vi "Setup.vi"(6 "Config in":T1, 7 "DisplayFilter":u8(ring)=7 items=["K_CHAN_R", "K_CHAN_W", "K_CHAN_RW", "K_CHAN_VOLT", "K_CHAN_FAULT", "K_ALL", "K_CUSTOM", "K_CHAN_R_VIS", "K_CHAN_W_VIS", "K_CHAN_RW_VIS", "K_CHAN_VOLT_VIS", "K_CHAN_FAULT_VIS"], 8 "error in (no error)":errorcluster, 9 "Caption":string, 10 "nodePath":string, 11 "NIVS.System Definition Root":refnum<k24>) -> (0 "error out":errorcluster, 1 "Caption out":string, 2 "Cancel?":bool, 3 "Selected Item":T2, 4 "List out":T1)   [LabVIEW 2015, in "Workspace.Obejct.Radio.lvlib"]
uses:
  Workspace.Obejct.Radio.lvlib
  NationalInstruments.VeriStand.SystemStorageUI
  NationalInstruments.VeriStand.SystemStorage
  <vilib>/NI Veristand/UI Controls/Single Node Browser/Node Ref.ctl
  Types/Config.ctl
  Types/Setup.StateVariables.ctl
  <vilib>/NI Veristand/UI Controls/Single Node Browser/Net Event Data.ctl
  <vilib>/NI Veristand/UI Controls/Single Node Browser/Net Event.ctl
  <vilib>/Utility/miscctls.llb/LVRowAndColumnTypeDef.ctl
  NationalInstruments.VeriStand
  <vilib>/NI Veristand/UI Controls/Single Node Browser/NI_VS UI Single Node Browser.lvlib
panel:
  in  "AutoUpdate":bool
  in  "Cancel":bool
  in  "OK":bool
  in  "Value":i64
  in  "Name":string
  in  "Text Value Pairing":i32(listbox)
  in  "Single Node Browser":refnum<k24>(container)
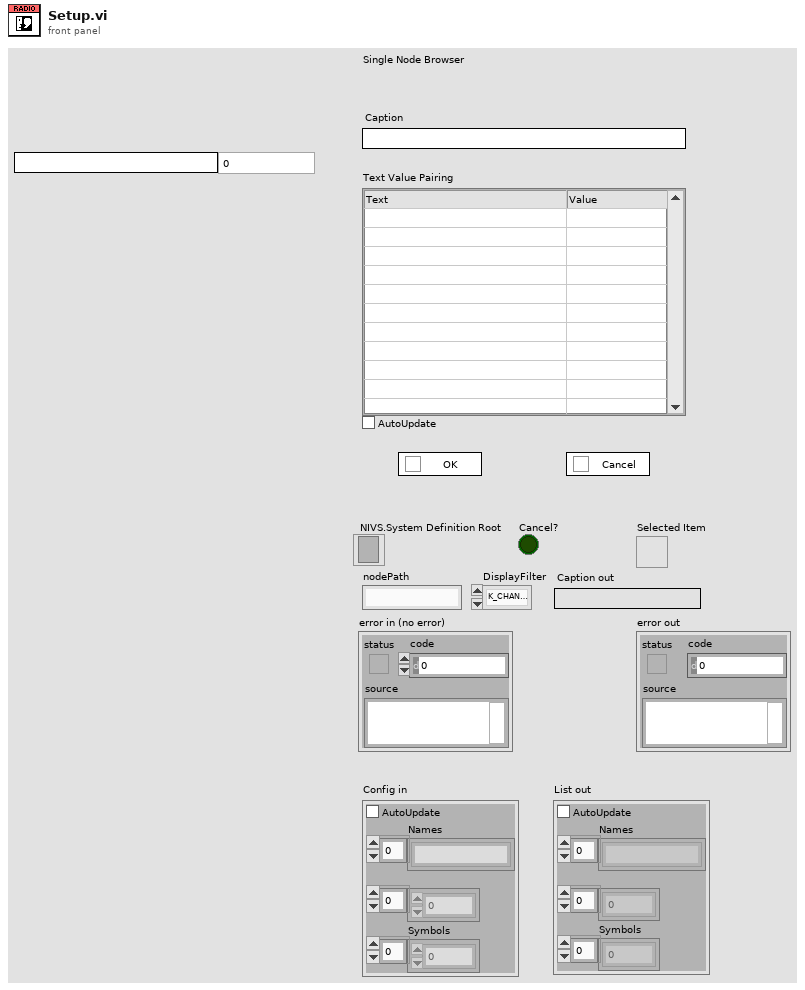
[diagram p1: front panel]
types:
  T1 = typedef "Workspace.Obejct.Radio.lvlib/Config.ctl" = cluster{"AutoUpdate":bool, "Names":string[], "Values":dbl[], "Symbols":i32[]}
  T2 = typedef "NI_VS UI Single Node Browser.lvlib/Node Ref.ctl" = refnum<k24>
  T3 = typedef "Workspace.Obejct.Radio.lvlib/Setup.StateVariables.ctl" = cluster{"UI.TextValuePairing":refnum<vi>, "UI.AutoUpdate":refnum<vi>, "UI.Name":refnum<vi>, "UI.Value":refnum<vi>, "UI.Caption":refnum<vi>, "UI.Events":refnum<event-registration>, "Config":T1, "NIVS.SystemDefinitionRoot":refnum<k24>, "NIVS.SingleNodeBrowser":refnum<k24>, "NIVS.NodePath":string, "NIVS.DisplayFilter":u8, "NIVS.Node":refnum<k24>, "Cache.Row":i32, "Cache.CellPosition":T4}
  T4 = typedef "LVRowAndColumnTypeDef.ctl" = cluster{"Row":i32, "Column":i32}
  T5 = enum8{"Enabled", "Disabled", "Disabled and Grayed Out"}
  T6 = typedef "LVPoint32TypeDef.ctl" = cluster{"Horizontal":i32, "Vertical":i32}
  T7 = typedef "LVPositionTypeDef.ctl" = cluster{"Left":i32, "Top":i32}
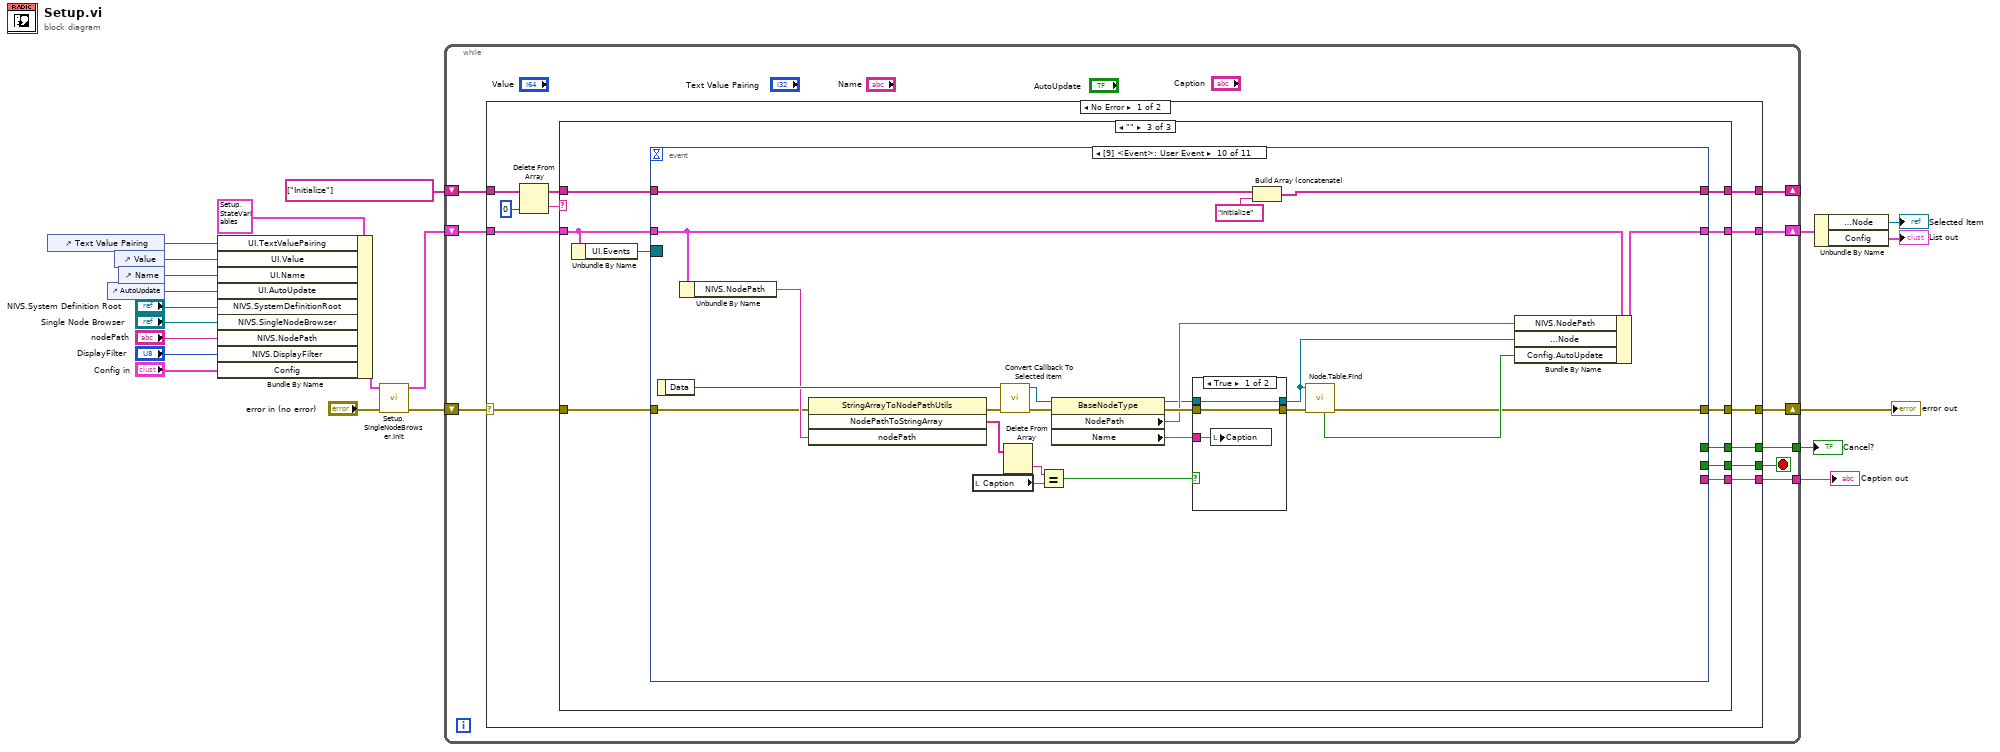
[diagram p0: block diagram]
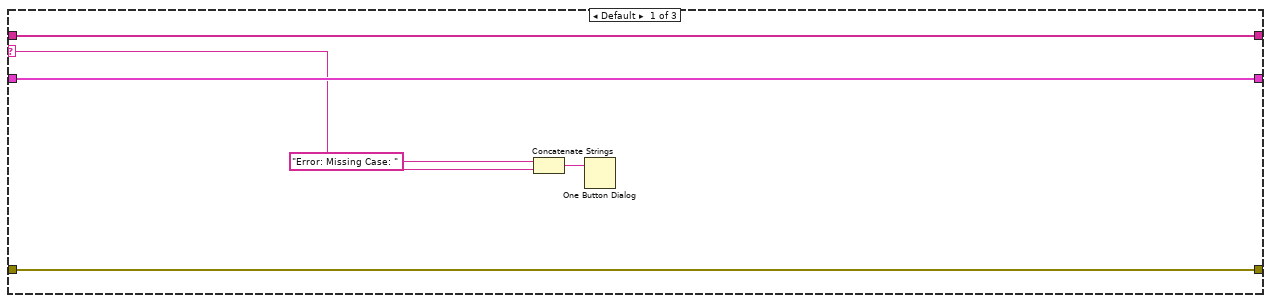
[diagram p2: hidden frame]
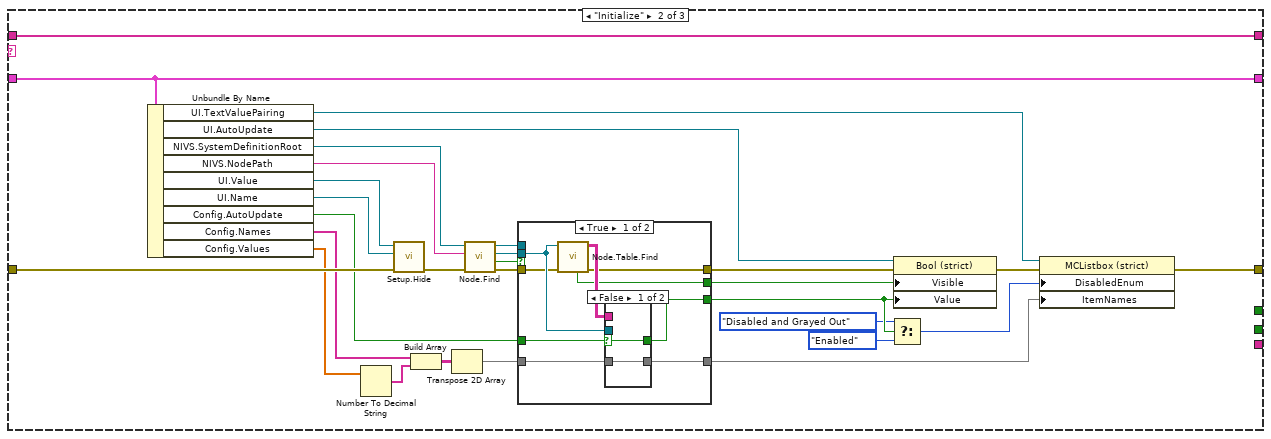
[diagram p3: hidden frame]
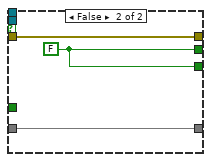
[diagram p5: hidden frame]
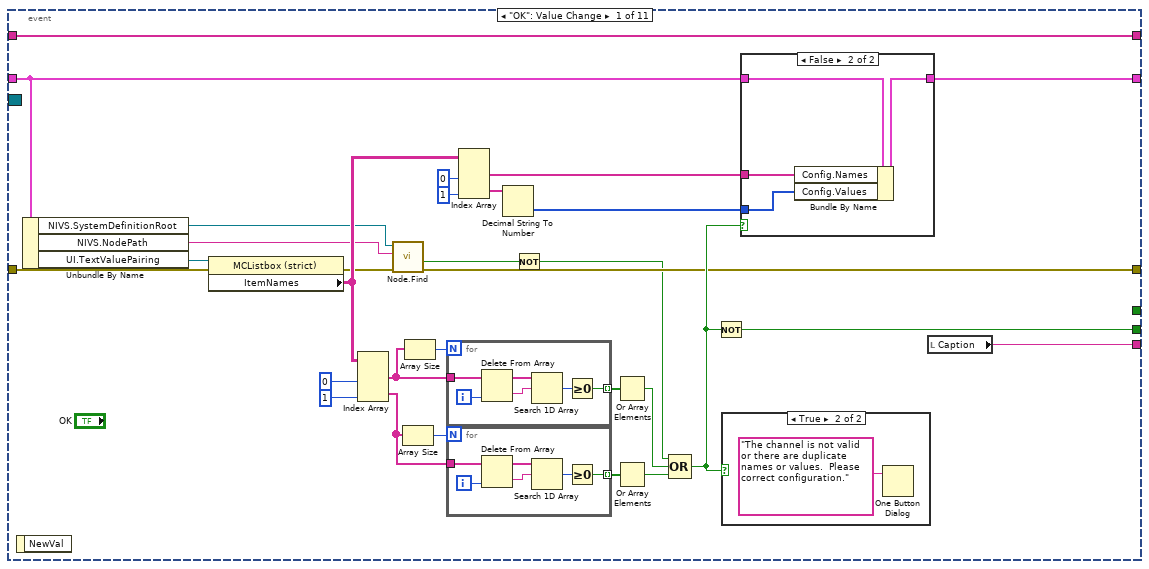
[diagram p6: hidden frame]
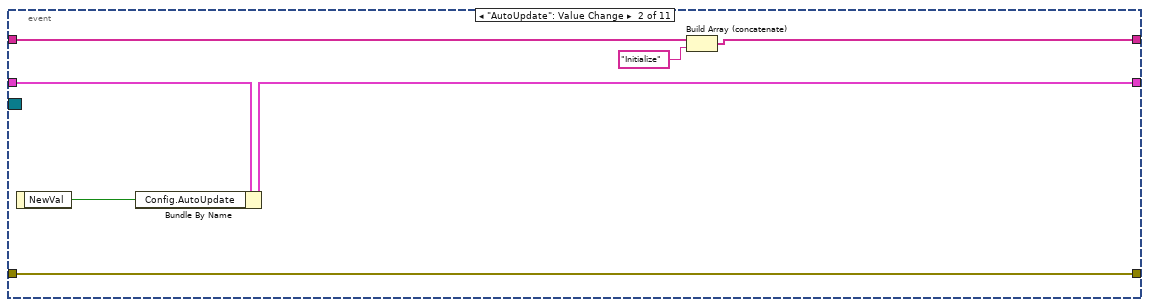
[diagram p9: hidden frame]
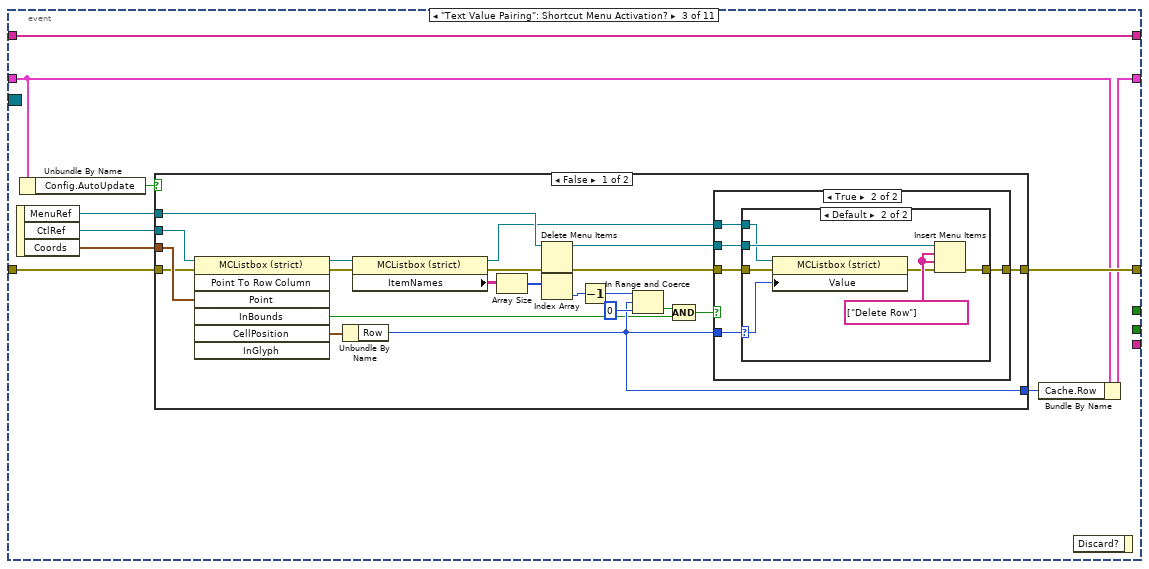
[diagram p10: hidden frame]
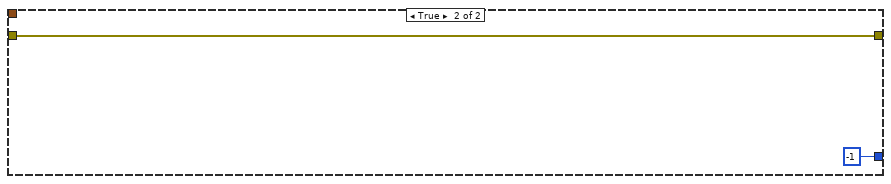
[diagram p13: hidden frame]
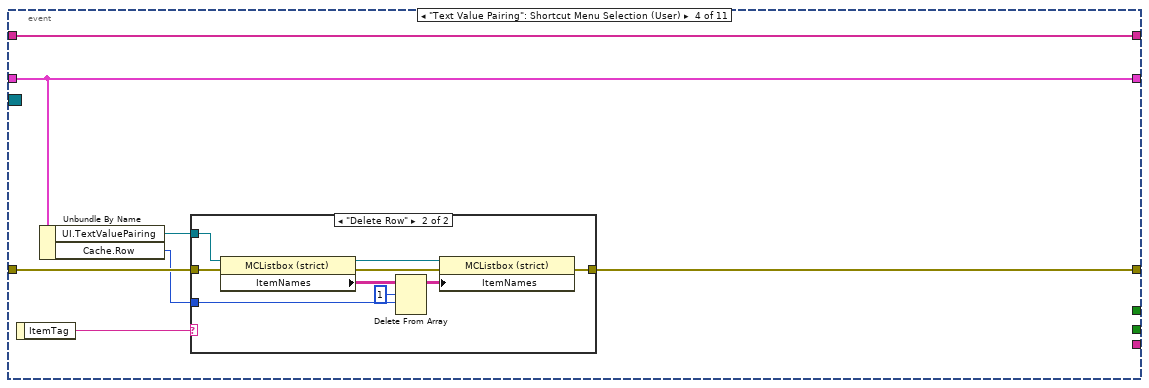
[diagram p14: hidden frame]
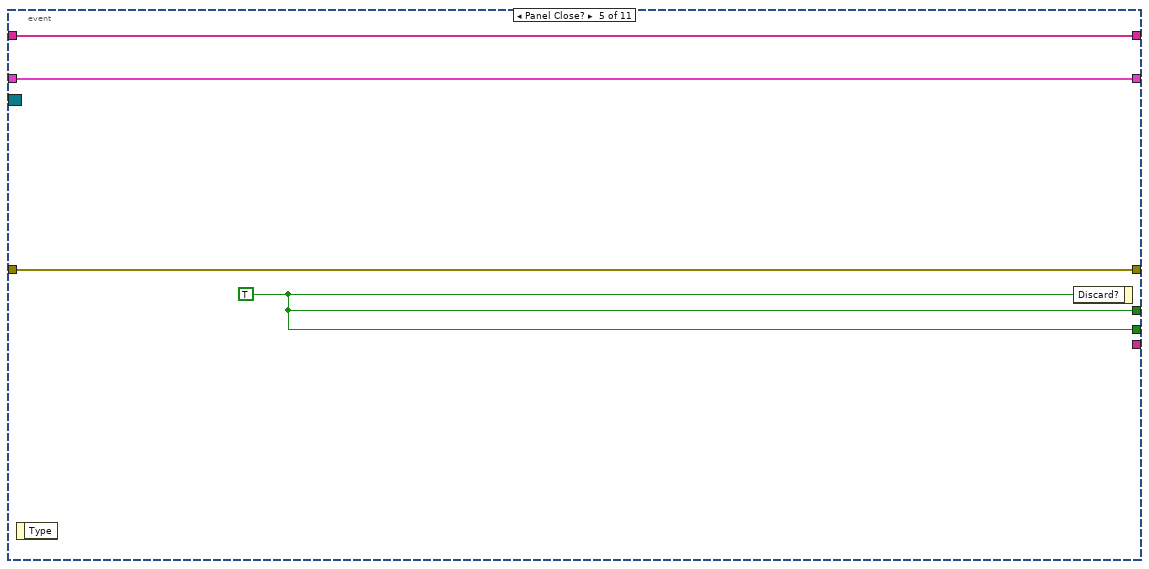
[diagram p16: hidden frame]
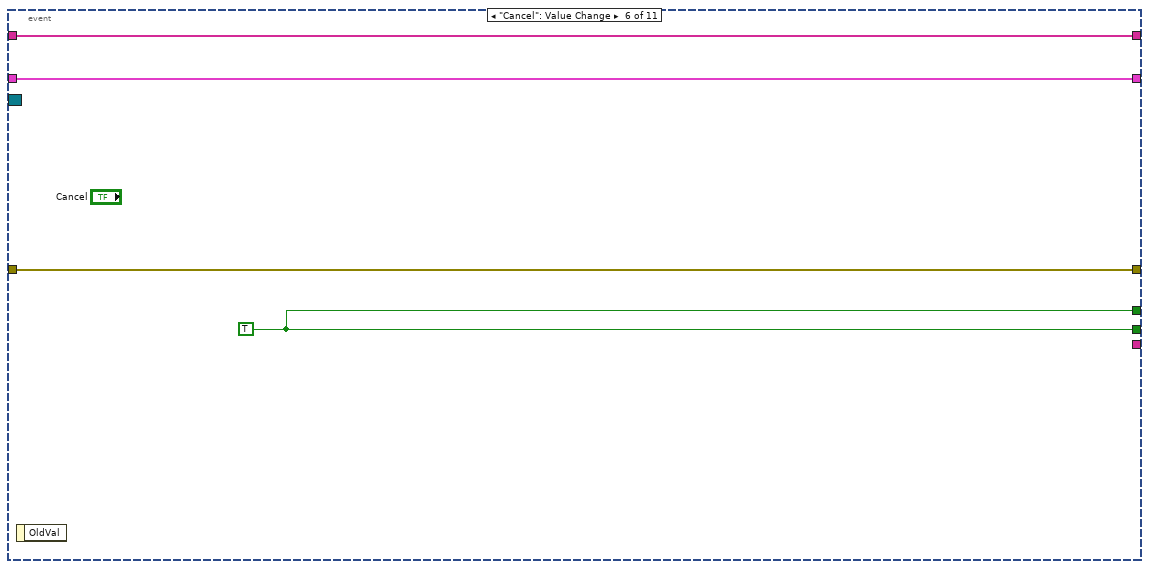
[diagram p17: hidden frame]
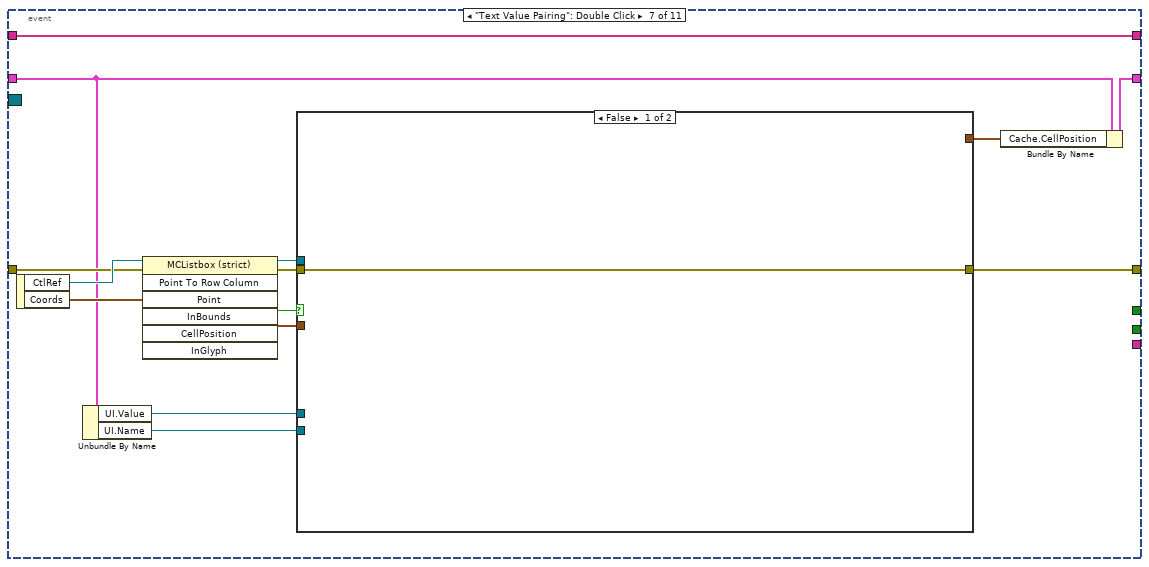
[diagram p18: hidden frame]
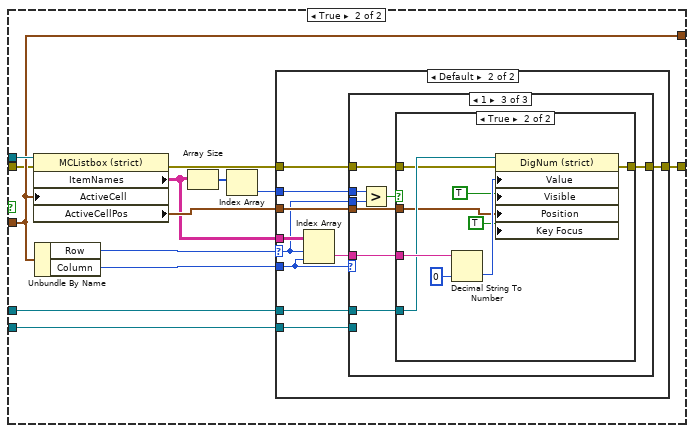
[diagram p19: hidden frame]
diagram:
  n1 = control-ref of="Text Value Pairing"() -> (w20:refnum<vi>)
  n2 = control-ref of="AutoUpdate"() -> (w17:refnum<vi>)
  n3 = control-ref of="Value"() -> (w19:refnum<vi>)
  n4 = control-ref of="Name"() -> (w18:refnum<vi>)
  n5 = Bundle By Name(cluster=T3 {"UI.TextValuePairing"=refnum, "UI.AutoUpdate"=refnum, "UI.Name"=refnum, "UI.Value"=refnum, "UI.Caption"=refnum, "UI.Events"=refnum, "Config"={"AutoUpdate"=FALSE, "Names"=[], "Values"=[], "Symbols"=[]}, "NIVS.SystemDefinitionRoot"=refnum, "NIVS.SingleNodeBrowser"=refnum, "NIVS.NodePath"="", "NIVS.DisplayFilter"=7, "NIVS.Node"=refnum, "Cache.Row"=0, "Cache.CellPosition"={"Row"=0, "Column"=0}} ("Cluster"), "UI.TextValuePairing"=w20, "UI.Value"=w19, "UI.Name"=w18, "UI.AutoUpdate"=w17, "NIVS.SystemDefinitionRoot"="NIVS.System Definition Root", "NIVS.SingleNodeBrowser"="Single Node Browser", "NIVS.NodePath"="nodePath", "NIVS.DisplayFilter"="DisplayFilter", "Config"="Config in") -> (w11:T3)
  n6 = call "Setup.SingleNodeBrowser.Init.vi"("error in (no error)"="error in (no error)", "Variables"=w11) -> ("error out"=w10:errorcluster, "Cluster out"=w9:T3)  [unwired: 8 in]
  n7 = while {
    shift-right: [w29] -> w5
    shift-left: w10 -> [w26]
    shift-right: [w27] -> w4
    shift-left: w9 -> [w28]
    shift-right: [w24] -> _
    shift-left: string[] ["Initialize"] -> [w25]
    tunnel: [w23] -> w6
    tunnel: [w22] -> w1
    stop <- w30 stop-if-true
    n8 = case shown="No Error" w26 {
      selector: w26 -> [w38 w399]
      tunnel: [w42 _] -> w30
      tunnel: [w41 w398] -> w29
      tunnel: w28 -> [w40 w402]
      tunnel: [w39 w402] -> w27
      tunnel: w25 -> [w36 w401]
      tunnel: [w33 w401] -> w24
      tunnel: [w32 _] -> w23
      tunnel: [w31 _] -> w22
      frame No Error {
        n9 = Delete From Array(array=w36, index=0) -> (deleted portion=w35:string, array with subset deleted=w34:string[])  [unwired: 1 in]
        n10 = case shown="\"\"" w35 {
          selector: w35 -> [w45 _ _]
          tunnel: [_ _ w102] -> w42
          tunnel: [w47 w60 w100] -> w41
          tunnel: w40 -> [w48 w50 w95]
          tunnel: [w48 w50 w99] -> w39
          tunnel: w38 -> [w47 w77 w103]
          tunnel: w34 -> [w46 w49 w97]
          tunnel: [w46 w49 w98] -> w33
          tunnel: [_ _ w101] -> w32
          tunnel: [_ _ w96] -> w31
          frame Default {
            n11 = Concatenate Strings("Error: Missing Case: " ("string"), w45) -> (w44:string)
            n12 = One Button Dialog(message=w44) -> ()  [unwired: 1 in, 1 out]
          }
          frame "Initialize" {
            n13 = Unbundle By Name(w50) -> ("UI.TextValuePairing"=w61:refnum<vi>, "UI.AutoUpdate"=w62:refnum<vi>, "NIVS.SystemDefinitionRoot"=w63:refnum<k24>, "NIVS.NodePath"=w64:string, "UI.Value"=w75:refnum<vi>, "UI.Name"=w76:refnum<vi>, "Config.AutoUpdate"=w53:bool, "Config.Names"=w51:string[], "Config.Values"=w52:dbl[])
            n14 = Number To Decimal String(number=w52) -> (decimal integer string=w70:string[])  [unwired: 1 in]
            n15 = call "Setup.Hide.vi"("error in (no error)"=w77, "Name"=w76, "Value"=w75) -> ("error out"=w67:errorcluster)  [unwired: 8 in]
            n16 = Build Array(w51, w70) -> (w69:string[][])
            n17 = Transpose 2D Array(2D array=w69) -> (transposed array=w68:string[][])
            n18 = call "Node.Find.vi"("error in (no error)"=w67, "nodePath"=w64, "System Def Root"=w63) -> ("error out"=w74:errorcluster, "FindNode"=w73:bool, "Node"=w72:refnum<k24>, "System Def Root"=w71:refnum<k24>)  [unwired: 5 in]
            n19 = case shown="True" w73 {
              tunnel: [w79 w91] -> w66
              tunnel: w71 -> [_ _]
              tunnel: w74 -> [w78 w91]
              tunnel: w72 -> [w82 _]
              tunnel: w53 -> [w84 _]
              tunnel: [w83 w93] -> w57
              tunnel: [w80 w93] -> w58
              tunnel: [w86 w92] -> w59
              tunnel: w68 -> [w85 w92]
              frame True {
                n20 = call "Node.Table.Find.vi"("error in (no error)"=w78, "Node"=w82) -> ("error out"=w79:errorcluster, "Items"=w81:string[][], "Found?"=w80:bool)  [unwired: 5 in, 2 out]
                n21 = case shown="False" w84 {
                  selector: w84 -> [w87 w90]
                  tunnel: w82 -> [_ _]
                  tunnel: [w88 w89] -> w86
                  tunnel: w85 -> [w88 _]
                  tunnel: [w87 w90] -> w83
                  tunnel: w81 -> [_ w89]
                  frame False {
                  }
                  frame True {
                  }
                }
              }
              frame False {
                w93 = FALSE ("AliasView")
              }
            }
            n22 = Select(t=T5."Disabled and Grayed Out" ("Disabled"), s=w57, f=T5."Enabled" ("Disabled")) -> (s? t:f=w54:T5)
            n23 = property class="Bool (strict)"(reference=w62, error in=w66, "Visible"=w58, "Value"=w57) -> (error out=w65:errorcluster)  [unwired: 1 out]
            n24 = property class="MCListbox (strict)"(reference=w61, error in=w65, "DisabledEnum"=w54, "ItemNames"=w59) -> (error out=w60:errorcluster)  [unwired: 1 out]
          }
          frame "" {
            n25 = Unbundle By Name(w95) -> ("UI.Events"=w94:refnum<event-registration>)
            n26 = event shown="[9] <Event>: User Event" {
              selector: w94 -> [_ _ _ _ _ _ _ _ _ _ _]
              dyn-events: _ -> [_ _ _ _ _ _ _ _ _ _ _]
              timeout: _ -> [_ _ _ _ _ _ _ _ _ _ _]
              tunnel: [w121 _ _ _ w226 w230 _ _ _ _ _] -> w102
              tunnel: w103 -> [w133 w155 w165 w211 w225 w229 w237 w324 w363 w375 w396]
              tunnel: [w108 w155 w168 w210 w225 w229 w238 w318 w353 w367 w397] -> w100
              tunnel: [_ _ _ _ w226 w230 _ _ _ _ _] -> w101
              tunnel: [w132 _ _ _ _ _ _ _ _ _ _] -> w96
              tunnel: [w112 w152 w159 w208 w224 w228 w234 w309 w351 w380 w394] -> w99
              tunnel: w95 -> [w113 w153 w161 w208 w224 w228 w233 w309 w351 w378 w394]
              tunnel: [w120 w157 w163 w209 w223 w227 w236 w310 w352 w366 w395] -> w98
              tunnel: w97 -> [w120 w158 w163 w209 w223 w227 w236 w310 w352 w381 w395]
              event "OK": Value Change {
                n27 = event-data() -> ()  [unwired: 1 in, 1 out]
                n28 = Unbundle By Name(w113) -> ("NIVS.SystemDefinitionRoot"=w106:refnum<k24>, "NIVS.NodePath"=w107:string, "UI.TextValuePairing"=w119:refnum<vi>)
                n29 = property class="MCListbox (strict)"(reference=w119, error in=w133) -> (error out=w109:errorcluster, "ItemNames"=w115:string[][])  [unwired: 1 out]
                n30 = Index Array(array=w115, index (col) #1=0 ("disabled index (col)"), index (col) #2=1 ("index (col)")) -> (element #1=w128:string[], element #2=w124:string[])  [unwired: 2 in]
                n31 = call "Node.Find.vi"("error in (no error)"=w109, "nodePath"=w107, "System Def Root"=w106) -> ("error out"=w108:errorcluster, "FindNode"=w105:bool)  [unwired: 5 in, 2 out]
                n32 = Array Size(array=w124) -> (size(s)=w125:i32)
                n33 = Array Size(array=w128) -> (size(s)=w129:i32)
                n34 = for {
                  N: w129 -> [_]
                  tunnel: w128 -> [w151]
                  tunnel: [w146] -> w127 mode=indexing
                  i -> [w150]
                  n35 = Delete From Array(array=w151, index=w150) -> (deleted portion=w148:string, array with subset deleted=w149:string[])  [unwired: 1 in]
                  n36 = Search 1D Array(1D array=w149, element=w148) -> (index of element=w147:i32)  [unwired: 1 in]
                  n37 = Greater Or Equal To 0?(x=w147) -> (x >= 0?=w146:bool)
                }
                n38 = for {
                  N: w125 -> [_]
                  tunnel: w124 -> [w145]
                  tunnel: [w140] -> w123 mode=indexing
                  i -> [w144]
                  n39 = Delete From Array(array=w145, index=w144) -> (deleted portion=w142:string, array with subset deleted=w143:string[])  [unwired: 1 in]
                  n40 = Search 1D Array(1D array=w143, element=w142) -> (index of element=w141:i32)  [unwired: 1 in]
                  n41 = Greater Or Equal To 0?(x=w141) -> (x >= 0?=w140:bool)
                }
                n42 = Index Array(array=w115, index (col) #1=0 ("disabled index (col)"), index (col) #2=1 ("index (col)")) -> (element #1=w110:string[], element #2=w116:string[])  [unwired: 2 in]
                n43 = Decimal String To Number(string=w116) -> (number=w111:i32[])  [unwired: 2 in, 1 out]
                n44 = Not(x=w105) -> (.not. x?=w104:bool)
                n45 = Or Array Elements(Boolean array=w127) -> (logical OR=w126:bool)
                n46 = Or Array Elements(Boolean array=w123) -> (logical OR=w122:bool)
                n47 = Compound Arithmetic op=OR(w104, w126, w122) -> (w114:bool)
                n48 = Not(x=w114) -> (.not. x?=w121:bool)
                n49 = case shown="True" w114 {
                  frame False {
                  }
                  frame True {
                    n50 = One Button Dialog(message="The channel is not valid or there are duplicate names or values.  Please correct configuration.") -> ()  [unwired: 1 in, 1 out]
                  }
                }
                n51 = case shown="False" w114 {
                  tunnel: w113 -> [w134 w138]
                  tunnel: [w134 w137] -> w112
                  tunnel: w111 -> [_ w136]
                  tunnel: w110 -> [_ w135]
                  frame True {
                  }
                  frame False {
                    n52 = Bundle By Name(cluster=w138, "Config.Names"=w135, "Config.Values"=w136) -> (w137:T3)
                  }
                }
                n53 = local read "Caption"() -> (w132:string)
              }
              event "AutoUpdate": Value Change {
                n54 = event-data() -> ("NewVal"=w154:bool)  [unwired: 1 in]
                n55 = Bundle By Name(cluster=w153, "Config.AutoUpdate"=w154) -> (w152:T3)
                n56 = Build Array (concatenate)(w158, "Initialize") -> (w157:string[])
              }
              event "Text Value Pairing": Shortcut Menu Activation? {
                n57 = event-data() -> ("MenuRef"=w164:refnum<k9>, "CtlRef"=w167:refnum<vi>, "Coords"=w166:T6)  [unwired: 1 in]
                n58 = Unbundle By Name(w161) -> ("Config.AutoUpdate"=w162:bool)
                n59 = case shown="False" w162 {
                  tunnel: [w189 w205] -> w168
                  tunnel: w167 -> [w188 _]
                  tunnel: w166 -> [w187 _]
                  tunnel: w165 -> [w186 w205]
                  tunnel: [w177 -1 ("Row")] -> w160
                  tunnel: w164 -> [w171 _]
                  frame False {
                    n60 = invoke class="MCListbox (strict)" method="Point To Row Column"(reference=w188, error in=w186, "Point"=w187) -> (reference out=w184:refnum<vi>, error out=w183:errorcluster, "InBounds"=w175:bool, "CellPosition"=w185:T4)  [unwired: 4 in, 3 out]
                    n61 = Unbundle By Name(w185) -> ("Row"=w177:i32)
                    n62 = property class="MCListbox (strict)"(reference=w184, error in=w183) -> (reference out=w169:refnum<vi>, error out=w173:errorcluster, "ItemNames"=w182:string[][])
                    n63 = Array Size(array=w182) -> (size(s)=w181:i32[])
                    n64 = Delete Menu Items(6:w173, 9:w171) -> (0:w172:errorcluster, 3:w170:refnum<k9>)  [unwired: 2 in]
                    n65 = Index Array(array=w181) -> (element=w180:i32)  [unwired: 1 in]
                    n66 = Decrement(x=w180) -> (x-1=w179:i32)
                    n67 = In Range and Coerce(upper limit=w179, x=w177, lower limit=0) -> (In Range?=w176:bool)  [unwired: 1 out]
                    n68 = Compound Arithmetic op=AND(w176, w175) -> (w174:bool)
                    n69 = case shown="True" w174 {
                      tunnel: w170 -> [_ w195]
                      tunnel: [w190 w194] -> w189
                      tunnel: w172 -> [w190 w193]
                      tunnel: w177 -> [_ w192]
                      tunnel: w169 -> [_ w191]
                      frame False {
                      }
                      frame True {
                        n70 = case shown="Default" w192 {
                          selector: w192 -> [_ w197]
                          tunnel: w195 -> [_ w201]
                          tunnel: [w196 w203] -> w194
                          tunnel: w193 -> [w196 w200]
                          tunnel: w191 -> [_ w198]
                          frame -1 {
                          }
                          frame Default {
                            w202 = string[] ["Delete Row"] ("item names")
                            n71 = property class="MCListbox (strict)"(reference=w198, error in=w200, "Value"=w197) -> (error out=w199:errorcluster)  [unwired: 1 out]
                            n72 = Insert Menu Items(6:w199, 7:w202, 8:w202, 9:w201) -> (0:w203:errorcluster)  [unwired: 2 in, 2 out]
                          }
                        }
                      }
                    }
                  }
                  frame True {
                  }
                }
                n73 = Bundle By Name(cluster=w161, "Cache.Row"=w160) -> (w159:T3)
                n74 = event-data() -> ()  [unwired: 2 in, 1 out]
              }
              event "Text Value Pairing": Shortcut Menu Selection (User) {
                n75 = event-data() -> ("ItemTag"=w212:string)  [unwired: 1 in]
                n76 = Unbundle By Name(w208) -> ("UI.TextValuePairing"=w206:refnum<vi>, "Cache.Row"=w207:i32)
                n77 = case shown="\"Delete Row\"" w212 {
                  tunnel: w211 -> [w213 w222]
                  tunnel: w207 -> [_ w216]
                  tunnel: [w213 w215] -> w210
                  tunnel: w206 -> [_ w214]
                  frame "False", Default {
                  }
                  frame "Delete Row" {
                    n78 = property class="MCListbox (strict)"(reference=w214, error in=w222) -> (reference out=w220:refnum<vi>, error out=w221:errorcluster, "ItemNames"=w219:string[][])
                    n79 = Delete From Array(array=w219, length=1, index (row)=w216) -> (array with subset deleted=w218:string[][])  [unwired: 1 in, 1 out]
                    n80 = property class="MCListbox (strict)"(reference=w220, error in=w221, "ItemNames"=w218) -> (error out=w215:errorcluster)  [unwired: 1 out]
                  }
                }
              }
              event Panel Close? {
                w226 = TRUE ("Discard?")
                n81 = event-data() -> ()  [unwired: 1 in, 1 out]
                n82 = event-data("Discard?"=w226) -> ()  [unwired: 1 in, 1 out]
              }
              event "Cancel": Value Change {
                w230 = TRUE ("Discard?")
                n83 = event-data() -> ()  [unwired: 1 in, 1 out]
              }
              event "Text Value Pairing": Double Click {
                n84 = event-data() -> ("CtlRef"=w244:refnum<vi>, "Coords"=w243:T6)  [unwired: 1 in]
                n85 = Unbundle By Name(w233) -> ("UI.Value"=w231:refnum<vi>, "UI.Name"=w232:refnum<vi>)
                n86 = invoke class="MCListbox (strict)" method="Point To Row Column"(reference=w244, error in=w237, "Point"=w243) -> (reference out=w242:refnum<vi>, error out=w239:errorcluster, "InBounds"=w240:bool, "CellPosition"=w241:T4)  [unwired: 4 in, 3 out]
                n87 = case shown="False" w240 {
                  tunnel: w241 -> [_ w254]
                  tunnel: w242 -> [_ w258]
                  tunnel: w231 -> [_ w257]
                  tunnel: w232 -> [_ w255]
                  tunnel: [_ w254] -> w235
                  tunnel: w239 -> [w245 w253]
                  tunnel: [w245 w251] -> w238
                  frame False {
                  }
                  frame True {
                    n88 = property class="MCListbox (strict)"(reference=w258, error in=w253, "ActiveCell"=w254) -> (error out=w252:errorcluster, "ItemNames"=w250:string[][], "ActiveCellPos"=w256:T7)  [unwired: 1 out]
                    n89 = Unbundle By Name(w254) -> ("Row"=w246:i32, "Column"=w248:i32)
                    n90 = Array Size(array=w250) -> (size(s)=w249:i32[])
                    n91 = Index Array(array=w249) -> (element=w247:i32)  [unwired: 1 in]
                    n92 = case shown="Default" w246 {
                      selector: w246 -> [_ w260]
                      tunnel: w257 -> [_ w268]
                      tunnel: w256 -> [_ w267]
                      tunnel: w255 -> [_ w266]
                      tunnel: w252 -> [w259 w265]
                      tunnel: [w259 w264] -> w251
                      tunnel: w250 -> [_ w263]
                      tunnel: w248 -> [_ w262]
                      tunnel: w247 -> [_ w261]
                      frame -1 {
                      }
                      frame Default {
                        n93 = Index Array(array=w263, index (row)=w260, index (col)=w262) -> (element=w269:string)
                        n94 = case shown="1" w262 {
                          tunnel: w269 -> [_ w276 w294]
                          tunnel: w267 -> [_ w277 w292]
                          tunnel: w268 -> [_ _ w293]
                          tunnel: w266 -> [_ w278 _]
                          tunnel: w265 -> [w270 w275 w291]
                          tunnel: [w270 w274 w290] -> w264
                          tunnel: w261 -> [_ w273 w289]
                          tunnel: w260 -> [_ w272 w288]
                          frame Default {
                          }
                          frame 0 {
                            n95 = Greater Or Equal?(x=w273, y=w272) -> (x >= y?=w271:bool)
                            n96 = case shown="True" w271 {
                              tunnel: w278 -> [_ w286]
                              tunnel: w277 -> [_ w285]
                              tunnel: w276 -> [_ w284]
                              tunnel: w275 -> [w279 w282]
                              tunnel: [w279 w280] -> w274
                              frame False {
                              }
                              frame True {
                                n97 = property class="Str"(reference=w286, error in=w282, "Value"=w284, "Visible"=TRUE, "Position"=w285, "Key Focus"=TRUE) -> (error out=w280:errorcluster)  [unwired: 1 out]
                              }
                            }
                          }
                          frame 1 {
                            n98 = Greater?(x=w289, y=w288) -> (0:w287:bool)
                            n99 = case shown="True" w287 {
                              tunnel: w294 -> [_ w304]
                              tunnel: w293 -> [_ w303]
                              tunnel: w292 -> [_ w300]
                              tunnel: w291 -> [w295 w298]
                              tunnel: [w295 w296] -> w290
                              frame False {
                              }
                              frame True {
                                n100 = Decimal String To Number(string=w304, default (0L)=i64 0 ("default (0 I32)")) -> (number=w302:i64)  [unwired: 1 in, 1 out]
                                n101 = property class="DigNum (strict)"(reference=w303, error in=w298, "Value"=w302, "Visible"=TRUE, "Position"=w300, "Key Focus"=TRUE) -> (error out=w296:errorcluster)  [unwired: 1 out]
                              }
                            }
                          }
                        }
                      }
                    }
                  }
                }
                n102 = Bundle By Name(cluster=w233, "Cache.CellPosition"=w235) -> (w234:T3)
              }
              event "Name": Value Change {
                n103 = event-data() -> ("NewVal"=w323:string)  [unwired: 1 in]
                n104 = Unbundle By Name(w309) -> ("UI.Value"=w305:refnum<vi>, "UI.Name"=w306:refnum<vi>, "Cache.CellPosition"=w307:T4, "UI.TextValuePairing"=w308:refnum<vi>)
                n105 = property class="MCListbox (strict)"(reference=w308, error in=w324) -> (reference out=w320:refnum<vi>, error out=w311:errorcluster, "ItemNames"=w315:string[][])
                n106 = Array Size(array=w315) -> (size(s)=w317:i32[])
                n107 = Unbundle By Name(w307) -> ("Row"=w314:i32, "Column"=w322:i32)
                n108 = Index Array(array=w317) -> (element=w316:i32)  [unwired: 1 in]
                n109 = Equal?(x=w314, y=w316) -> (x = y?=w313:bool)
                n110 = case shown="True" w313 {
                  tunnel: w323 -> [w330 w333]
                  tunnel: w322 -> [w329 _]
                  tunnel: [w328 w340] -> w321
                  tunnel: w315 -> [w327 w339]
                  tunnel: w314 -> [w326 w338]
                  tunnel: [w325 w332] -> w312
                  tunnel: w311 -> [w325 w332]
                  frame False {
                    n111 = Replace Array Subset(array=w327, new element=w330, index (row)=w326, index (col)=w329) -> (w328:string[][])
                  }
                  frame True {
                    n112 = Decrement(x=w338) -> (x-1=w337:i32)
                    n113 = Index Array(array=w339, index (row)=w337, index (col)=1 ("disabled index (col)")) -> (element=w335:string)
                    n114 = case shown="Default" w335 {
                      selector: w335 -> [_ w344]
                      tunnel: [w341 w343] -> w334
                      frame "" {
                        n115 = Number To Decimal String(number=0) -> (decimal integer string=w341:string)  [unwired: 1 in]
                      }
                      frame Default {
                        n116 = Decimal String To Number(string=w344) -> (number=w345:i32)  [unwired: 2 in, 1 out]
                        n117 = Increment(x=w345) -> (x+1=w346:i32)
                        n118 = Number To Decimal String(number=w346) -> (decimal integer string=w343:string)  [unwired: 1 in]
                      }
                    }
                    n119 = Build Array(w333, w334) -> (w331:string[])
                    n120 = Build Array (concatenate)(w339, w331) -> (w340:string[][])
                  }
                }
                n121 = property class="MCListbox (strict)"(reference=w320, error in=w312, "ItemNames"=w321) -> (error out=w319:errorcluster)  [unwired: 1 out]
                n122 = call "Setup.Hide.vi"("error in (no error)"=w319, "Name"=w306, "Value"=w305) -> ("error out"=w318:errorcluster)  [unwired: 8 in]
              }
              event "Value": Value Change {
                n123 = event-data() -> ("NewVal"=w361:i64)  [unwired: 1 in]
                n124 = Unbundle By Name(w351) -> ("UI.Value"=w349:refnum<vi>, "UI.Name"=w350:refnum<vi>, "UI.TextValuePairing"=w348:refnum<vi>, "Cache.CellPosition"=w347:T4)
                n125 = property class="MCListbox (strict)"(reference=w348, error in=w363) -> (reference out=w356:refnum<vi>, error out=w358:errorcluster, "ItemNames"=w362:string[][])
                n126 = Unbundle By Name(w347) -> ("Row"=w360:i32, "Column"=w359:i32)
                n127 = Number To Decimal String(number=w361) -> (decimal integer string=w355:string)  [unwired: 1 in]
                n128 = Replace Array Subset(array=w362, new element=w355, index (row)=w360, index (col)=w359) -> (w357:string[][])
                n129 = property class="MCListbox (strict)"(reference=w356, error in=w358, "ItemNames"=w357) -> (error out=w354:errorcluster)  [unwired: 1 out]
                n130 = call "Setup.Hide.vi"("error in (no error)"=w354, "Name"=w350, "Value"=w349) -> ("error out"=w353:errorcluster)  [unwired: 8 in]
              }
              event User Event {
                n131 = event-data() -> ("Data"=w386:variant)  [unwired: 1 in]
                n132 = Unbundle By Name(w378) -> ("NIVS.NodePath"=w376:string)
                n133 = invoke class="StringArrayToNodePathUtils" method="NodePathToStringArray"(error in=w375, "nodePath"=w376) -> (error out=w374:errorcluster, "NodePathToStringArray"=w373:string[])  [unwired: 2 in, 2 out]
                n134 = local read "Caption"() -> (w371:string)
                n135 = call <vilib>:"Convert Callback To Selected Item.vi"("error in"=w374, "Data"=w386) -> ("error out"=w384:errorcluster, "Selected Item"=w385:T2)  [unwired: 8 in]
                n136 = Delete From Array(array=w373) -> (deleted portion=w372:string)  [unwired: 2 in, 1 out]
                n137 = Equal?(x=w372, y=w371) -> (x = y?=w370:bool)
                n138 = property class="BaseNodeType"(reference=w385, error in=w384) -> (reference out=w364:T2, error out=w383:errorcluster, "NodePath"=w368:string, "Name"=w369:string)
                n139 = case shown="True" w370 {
                  tunnel: w369 -> [w389 _]
                  tunnel: [w388 w391] -> w382
                  tunnel: w383 -> [w388 w391]
                  tunnel: [w387 w390] -> w379
                  tunnel: w364 -> [w387 w390]
                  frame True {
                    n140 = local write "Caption"(w389) -> ()
                  }
                  frame False {
                  }
                }
                n141 = Build Array (concatenate)(w381, "Initialize") -> (w366:string[])
                n142 = call "Node.Table.Find.vi"("error in (no error)"=w382, "Node"=w379) -> ("error out"=w367:errorcluster, "Found?"=w377:bool)  [unwired: 5 in, 3 out]
                n143 = Bundle By Name(cluster=w378, "NIVS.NodePath"=w368, "NIVS.Node"=w379, "Config.AutoUpdate"=w377) -> (w380:T3)
              }
              event "Value", "Name": Mouse Leave {
                n144 = event-data() -> ()  [unwired: 1 in, 1 out]
                n145 = Unbundle By Name(w394) -> ("UI.Value"=w393:refnum<vi>, "UI.Name"=w392:refnum<vi>)
                n146 = call "Setup.Hide.vi"("error in (no error)"=w396, "Name"=w392, "Value"=w393) -> ("error out"=w397:errorcluster)  [unwired: 8 in]
              }
            }
          }
        }
      }
      frame Error {
        n147 = call <vilib>:"Simple Error Handler.vi"("error in (no error)"=w399) -> ("error out"=w400:errorcluster)  [unwired: 4 in, 4 out]
        n148 = call <vilib>:"Clear Errors.vi"("error in (no error)"=w400) -> ("error out"=w398:errorcluster)  [unwired: 5 in, 1 out]
      }
    }
  }
  "error out" <- w5
  "Cancel?" <- w6
  "Caption out" <- w1
  n149 = Unbundle By Name(w4) -> ("NIVS.Node"=→"Selected Item":refnum<k24>, "Config"=→"List out":T1)
